vi "TrapProfState_New.vi"(9 "Velocity":dbl format="%20.4f", 11 "Position":dbl format="%20.4f") -> (3 "TRAPEZOID_PROFILE_STATE":T1 {"Velocity" format="%16_6e"; "Position" format="%16_6e"})   [LabVIEW 2019, in "Trajectory_Library.lvlib"]
doc: "Creates a new Trapzoid Profile State data cluster. This could be a demand, actual, or goal (setpoint) data cluster depending on how it is used.\n\nInputs:\n - Position -- Value for position\n - Velocity -- Value for velocity.\n\nOutputs::\n - Trapezoid_Profile_State -- Initialized data cluster"
uses:
  Trajectory_Library.lvlib
  TRAPEZOID_PROFILE_STATE.ctl
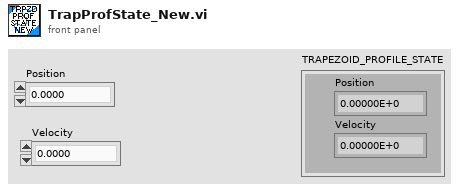
[diagram p1: front panel]
types:
  T1 = typedef "Trajectory_Library.lvlib/TRAPEZOID_PROFILE_STATE.ctl" = cluster{"Position":dbl, "Velocity":dbl}
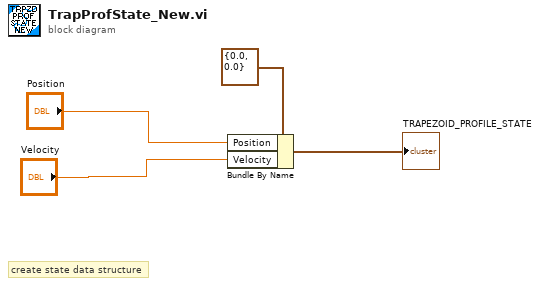
[diagram p0: block diagram]
diagram:
  # "create state data structure"
  n1 = Bundle By Name(cluster=T1 {"Position"=0.0, "Velocity"=0.0} ("TRAPEZOID_PROFILE_STATE"), "Position"="Position", "Velocity"="Velocity") -> (→"TRAPEZOID_PROFILE_STATE":T1)
